vi "Timer.vi"(0 "Wait_Time":i32=10, 11 "Error_In":errorcluster, 13 "Timer_Select":T1=enum."Time_Out?") -> (4 "Time_Out?":bool, 6 "Time":dbl, 15 "Error_Out":errorcluster)   [LabVIEW 2021]
doc: "This is the timer vi that works as a typical timer.\nStart to start the timer.\nif timer paused, again start the timer and check for time out?."
uses:
  Control/Timer_Data.ctl
  Control/Timer_Operation_Select.ctl
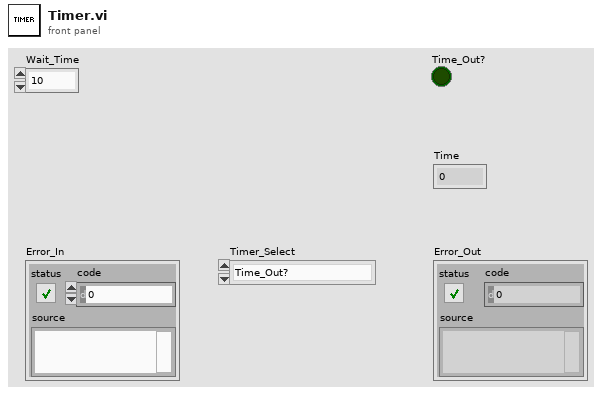
[diagram p1: front panel]
types:
  T1 = typedef "Timer_Operation_Select.ctl" = enum16{"Start_Timer", "Pause_Timer", "Time_Out?", "Stop_Timer"}
  T2 = typedef "Timer_Data.ctl" = cluster{"Start_Time":dbl, "Start?":bool, "Wait_Time":dbl, "Pause_Time":dbl, "Time":dbl}
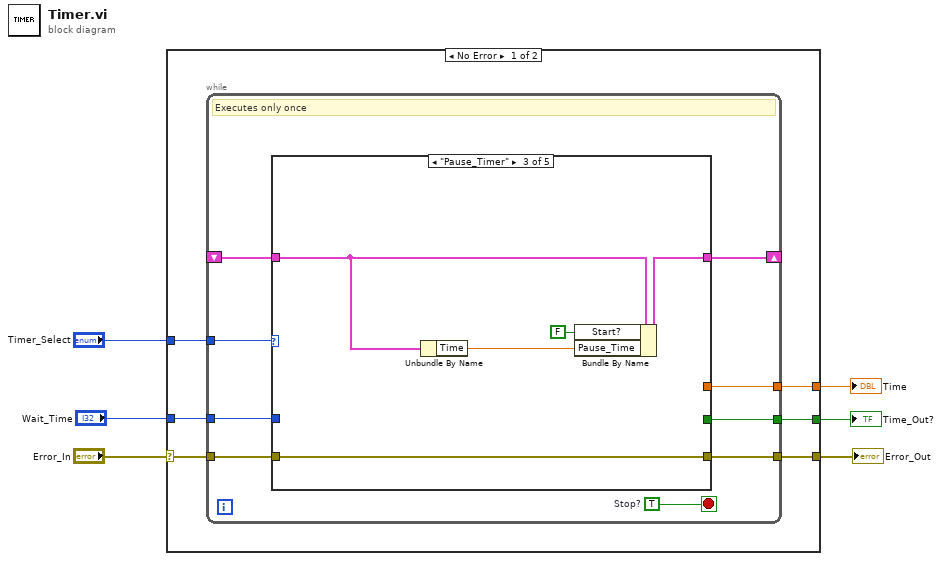
[diagram p0: block diagram]
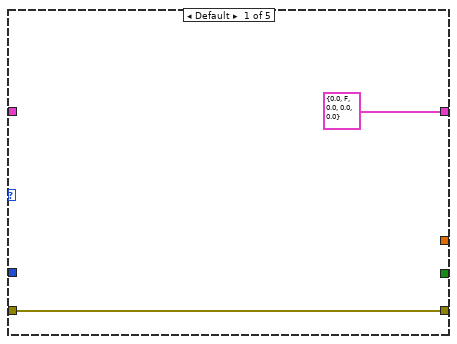
[diagram p2: hidden frame]
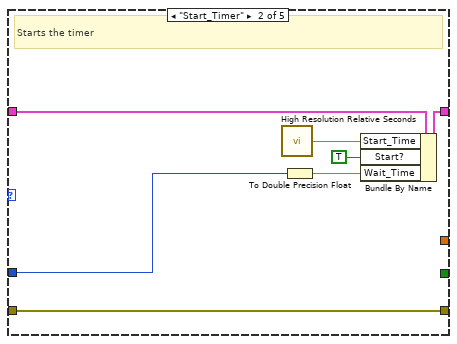
[diagram p3: hidden frame]
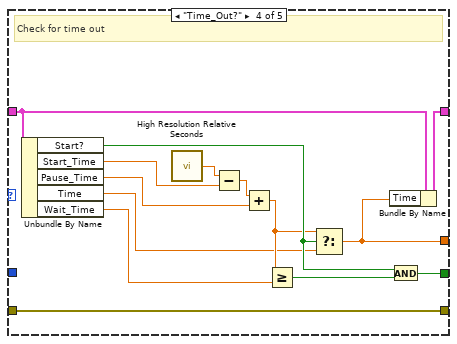
[diagram p4: hidden frame]
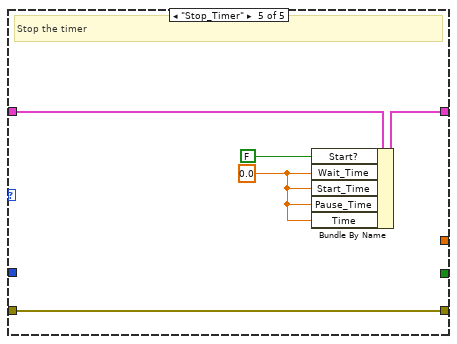
[diagram p5: hidden frame]
diagram:
  n1 = case shown="No Error" "Error_In" {
    selector: "Error_In" -> [w8 w55]
    tunnel: [w12 _] -> w6
    tunnel: [w11 w55] -> w5
    tunnel: "Wait_Time" -> [w10 _]
    tunnel: "Timer_Select" -> [w9 _]
    tunnel: [w7 _] -> w1
    frame No Error {
      n2 = while {
        tunnel: w9 -> [w21]
        shift-right: [w20] -> _
        shift-left: _ -> [w19]
        tunnel: [w18] -> w12
        tunnel: w8 -> [w16]
        tunnel: [w15] -> w11
        tunnel: w10 -> [w14]
        tunnel: [w13] -> w7
        stop <- w17 stop-if-true
        w17 = TRUE  # Stop?
        # "Executes only once"
        n3 = case shown="\"Pause_Timer\"" w21 {
          tunnel: [T2 {"Start_Time"=0.0, "Start?"=FALSE, "Wait_Time"=0.0, "Pause_Time"=0.0, "Time"=0.0} ("Cluster") w28 w35 w40 w52] -> w20
          tunnel: w19 -> [_ w29 w32 w45 w53]
          tunnel: [_ _ _ w46 _] -> w18
          tunnel: w16 -> [w23 w30 w34 w48 w54]
          tunnel: [w23 w30 w34 w48 w54] -> w15
          tunnel: w14 -> [_ w25 _ _ _]
          tunnel: [_ _ _ w36 _] -> w13
          frame Default {
          }
          frame "Start_Timer" {
            # "Starts the timer"
            n4 = call <vilib>:"High Resolution Relative Seconds.vi"() -> ("relative seconds"=w27:dbl)
            n5 = To Double Precision Float(number=w25) -> (double precision float=w24:dbl)
            n6 = Bundle By Name(cluster=w29, "Start_Time"=w27, "Start?"=TRUE, "Wait_Time"=w24) -> (w28:T2)
          }
          frame "Pause_Timer" {
            n7 = Unbundle By Name(w32) -> ("Time"=w31:dbl)
            n8 = Bundle By Name(cluster=w32, "Start?"=FALSE, "Pause_Time"=w31) -> (w35:T2)
          }
          frame "Time_Out?" {
            # "Check for time out"
            n9 = Unbundle By Name(w45) -> ("Start?"=w41:bool, "Start_Time"=w44:dbl, "Pause_Time"=w42:dbl, "Time"=w37:dbl, "Wait_Time"=w38:dbl)
            n10 = call <vilib>:"High Resolution Relative Seconds.vi"() -> ("relative seconds"=w47:dbl)
            n11 = Subtract(x=w47, y=w44) -> (x-y=w43:dbl)
            n12 = Add(x=w43, y=w42) -> (x+y=w39:dbl)
            n13 = Greater Or Equal?(x=w39, y=w38) -> (x >= y?=w49:bool)
            n14 = Select(t=w39, s=w41, f=w37) -> (s? t:f=w36:dbl)
            n15 = Bundle By Name(cluster=w45, "Time"=w36) -> (w40:T2)
            n16 = And(x=w41, y=w49) -> (x .and. y?=w46:bool)
          }
          frame "Stop_Timer" {
            w50 = 0.0 ("Wait_Time")
            # "Stop the timer"
            n17 = Bundle By Name(cluster=w53, "Start?"=FALSE, "Wait_Time"=w50, "Start_Time"=w50, "Pause_Time"=w50, "Time"=w50) -> (w52:T2)
          }
        }
      }
    }
    frame Error {
    }
  }
  "Time_Out?" <- w6
  "Error_Out" <- w5
  "Time" <- w1
